vi "Plot Editor Asynchronous Call.vi"(8 "error in (no error)":errorcluster, 10 "Coords":T1, 11 "XYGraph in":T2) -> (0 "Error Out":errorcluster, 1 "Message":string, 2 "Plot Name":string, 3 "Graph Name":string)   [LabVIEW 2021, in "Plot Editor.lvlib"]
uses:
  Plot Editor.lvlib
  XY Graph/XY Graph Refnum.ctl
  <vilib>/Utility/miscctls.llb/LVPoint32TypeDef.ctl
  Get Plot at Mouse Click (XY Graph)/Get Plot at Mouse Click [AAC].vi
  Graphs.lvlib
  XY Graph/XY Graph Add-Ons.lvlib
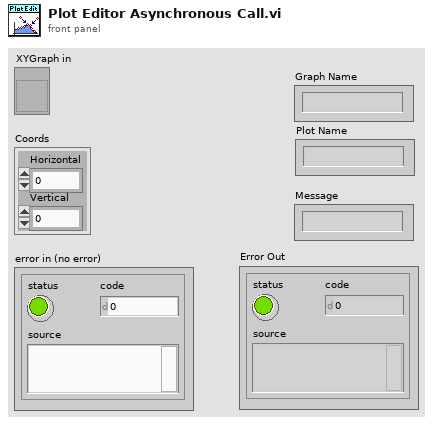
[diagram p1: front panel]
types:
  T1 = typedef "LVPoint32TypeDef.ctl" = cluster{"Horizontal":i32, "Vertical":i32}
  T2 = typedef "XY Graph Add-Ons.lvlib/XY Graph Refnum.ctl" = refnum<vi>
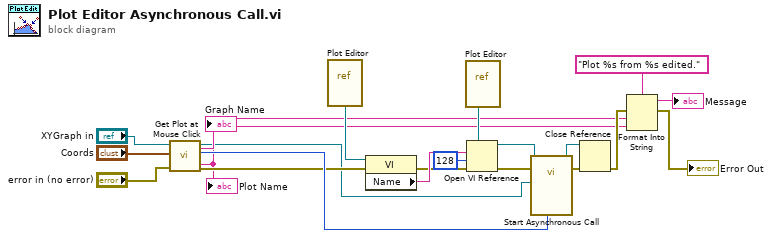
[diagram p0: block diagram]
diagram:
  n1 = call-poly "Get Plot at Mouse Click.vi"("error in (no error)"="error in (no error)", "Mouse Click Coordinates"="Coords", "XYGraph Ref"="XYGraph in") -> ("error out"=w17:errorcluster, "Plot at Coordinates"=w21:i32, "XYGraph Ref"=w2:T2, "Plot Name"=w3:string, "Graph Name"=w4:string)  [unwired: 2 in, 2 out]
  "Plot Name" <- w3
  "Graph Name" <- w4
  n2 = vi-ref "Plot Editor.vi"() -> (w9:refnum<vi>)
  n3 = property class="VI"(reference=w9, error in=w17) -> (error out=w10:errorcluster, "Name"=w11:string)  [unwired: 1 out]
  n4 = vi-ref "Plot Editor.vi"() -> (w12:refnum<vi>)
  n5 = Open VI Reference(type specifier VI Refnum (for type only)=w12, vi path=w11, options=128, error in (no error)=w10) -> (vi reference=w15:refnum<vi>, error out=w16:errorcluster)  [unwired: 2 in]
  n6 = call-by-ref "Start Asynchronous Call"(reference=w15, error in=w16, "Original Plot Idx"=w21, "Original Graph Refnum"=w2) -> (reference out=w14:refnum<vi>, error out=w13:errorcluster)  [unwired: 7 in, 3 out]
  n7 = Close Reference(reference=w14, error in (no error)=w13) -> (error out=w7:errorcluster)
  n8 = Format Into String(format string="Plot %s from %s edited.", error in=w7, w3, w4) -> (resulting string=→"Message":string, error out=→"Error Out":errorcluster)  [unwired: 1 in]
